vi "chart1.vi"(7 "LabVIEW Web Service Request":refnum<class "Web Request.lvclass">) -> ()   [LabVIEW 2019]
uses:
  <vilib>/wsapi/Web Request.lvclass
panel:
  out "error out":errorcluster
  in  "error in (no error)":errorcluster
  in  "Stop Button":bool
  out "Waveform Chart":dbl(graph)
  # "Use the Web Service Request input terminal to call the VIs on the Web Services palette. Do not remove it from the connector pane unless you don't need access to the palette."
  # "Each additional control wired to the connector pane will be available as an input in the URL. To include an indicator in terminal-mode output (the default setting), it must also be wired to the connector pane."
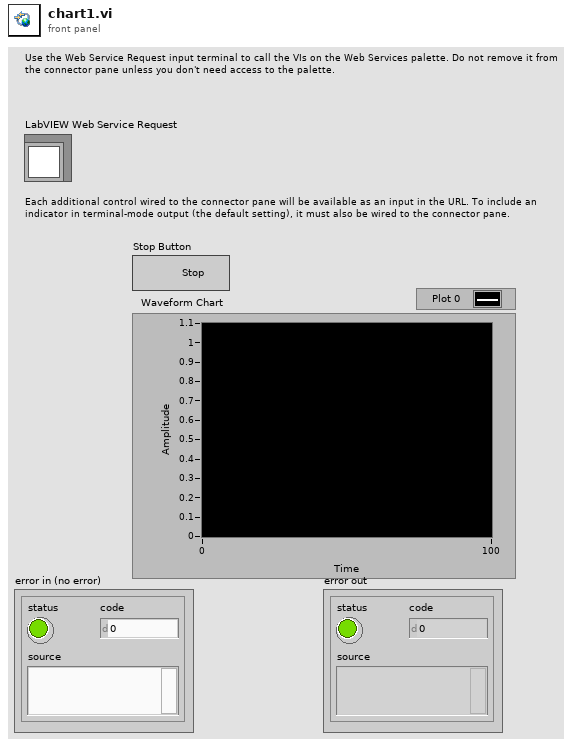
[diagram p1: front panel]
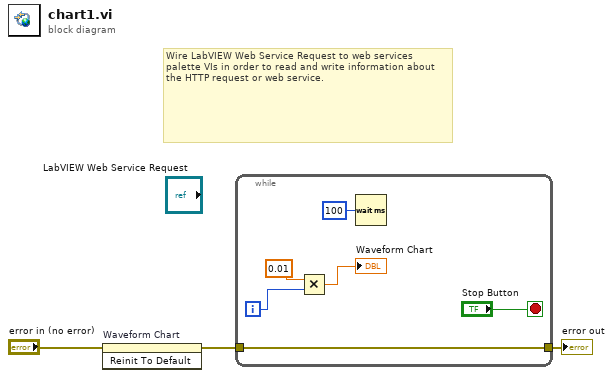
[diagram p0: block diagram]
diagram:
  # "Wire LabVIEW Web Service Request to web services palette VIs in order to read and write information about the HTTP request or web service."
  n1 = invoke on="Waveform Chart" class="WFChart (strict)" method="Reinit To Default"(error in="error in (no error)") -> (error out=w2:errorcluster)  [unwired: 2 in, 2 out]
  n2 = while {
    tunnel: w2 -> [w4]
    tunnel: [w4] -> w1
    i -> [w9]
    stop <- "Stop Button" stop-if-true
    n3 = Multiply(x=0.01, y=w9) -> (x*y=→"Waveform Chart":dbl)
    n4 = Wait (ms)(milliseconds to wait=u32 100) -> ()  [unwired: 1 out]
  }
  "error out" <- w1
